vi "initial.vi"(8 "error in (no error)":errorcluster, 11 "ZanCard in":refnum<class "ZanCard.lvclass">) -> (0 "error out":errorcluster, 3 "ZanCard out":refnum<class "ZanCard.lvclass">)   [LabVIEW 2019, in "ZanCard.lvclass"]
uses:
  ZanCard.lvclass
  IOCard.lvclass/IOCard.ctl
  ZanCard.lvclass/ZanCard.ctl
  LLB/zmotion/zaux/zauxdll.lvlib
  IOCard.lvclass
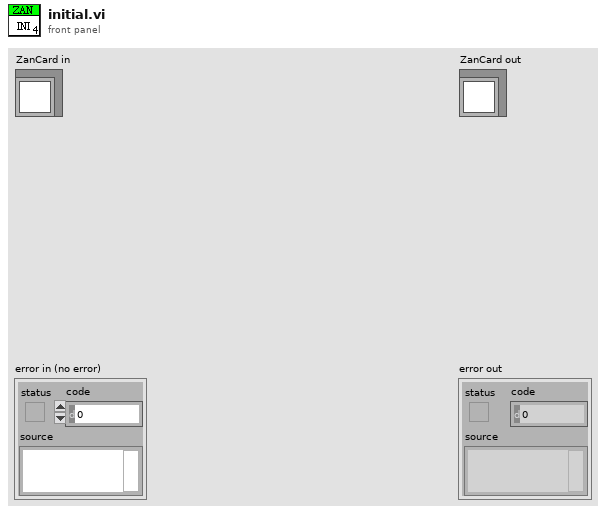
[diagram p1: front panel]
types:
  T1 = typedef "IO Card_Type.ctl" = enum16{"None", "Unidaq32", "6480", "2410C-64", "Zan", "DMC1000B", "16InOut", "Robot", "DMC3600"}
  T2 = cluster{"IO Card Type":T1, "IOType":enum16{"Input", "Output"}, "CardNumber":i32, "ConnectAct":bool, "IP":string}
  T3 = cluster{"CardNumber":i32, "Connect":bool, "Handler":i32}
  T4 = cluster{"Card":i32, "Connect":bool, "Handler":i32}[]
  T5 = cluster{"Card":i32, "Connect":bool, "Handler":i32}
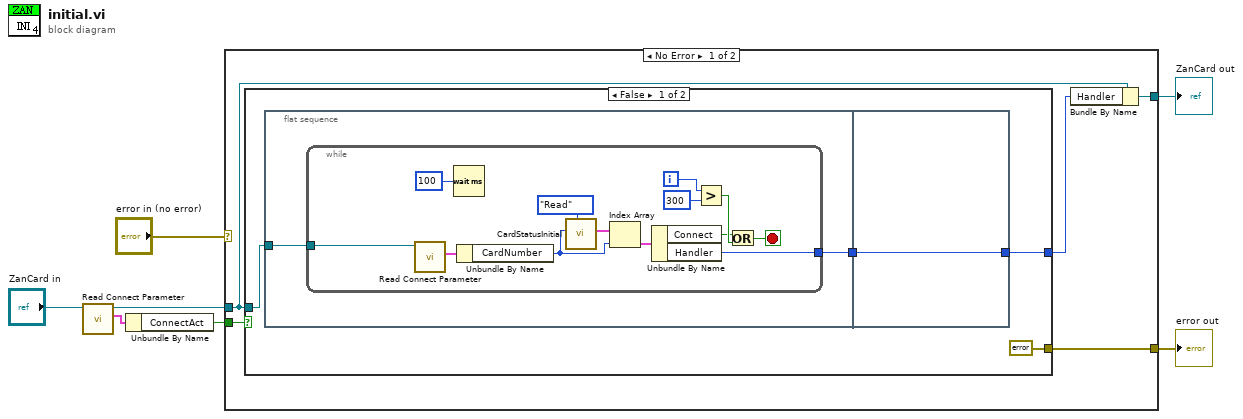
[diagram p0: block diagram]
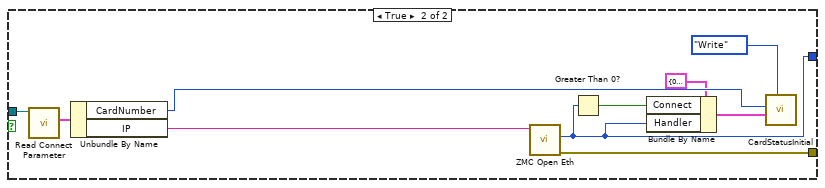
[diagram p2: hidden frame]
diagram:
  n1 = call "Read Connect Parameter.vi"("IOCard in"="ZanCard in") -> ("Connect Parameter"=w2:T2, "IOCard out"=w3:refnum<class "ZanCard.lvclass">)  [unwired: 8 in, 1 out]
  n2 = Unbundle By Name(w2) -> ("ConnectAct"=w1:bool)
  n3 = case shown="No Error" "error in (no error)" {
    selector: "error in (no error)" -> [_ w44]
    tunnel: [w12 w44] -> w6
    tunnel: w3 -> [w9 w43]
    tunnel: [w11 w43] -> w5
    tunnel: w1 -> [w8 _]
    frame No Error {
      n4 = case shown="False" w8 {
        tunnel: [errorcluster {"status"=FALSE, "code"=0, "source"=""} ("error out") w42] -> w12
        tunnel: w9 -> [w14 w41]
        tunnel: [w15 w33] -> w10
        frame False {
          n5 = flat-sequence {
            tunnel: w14 -> [w18]
            tunnel: [w17] -> w13
            tunnel: [w32] -> w15
            tunnel: w13 -> [w32]
            frame #0 {
              n6 = while {
                tunnel: w18 -> [w25]
                tunnel: [w19] -> w17
                i -> [w29]
                stop <- w30 stop-if-true
                n7 = call "Read Connect Parameter.vi"("IOCard in"=w25) -> ("Connect Parameter"=w24:T2)  [unwired: 8 in, 2 out]
                n8 = Wait (ms)(milliseconds to wait=u32 100) -> ()  [unwired: 1 out]
                n9 = Unbundle By Name(w24) -> ("CardNumber"=w22:i32)
                n10 = call "CardStatusInitial.vi"("Action"=enum16{"Initial", "Write", "Read", "Release"}."Read", "CardNumber"=w22) -> ("CardStatus"=w23:T4)  [unwired: 9 in]
                n11 = Index Array(array=w23, index=w22) -> (element=w21:T5)
                n12 = Unbundle By Name(w21) -> ("Connect"=w20:bool, "Handler"=w19:i32)
                n13 = Greater?(x=w29, y=300) -> (0:w27:bool)
                n14 = Or(x=w20, y=w27) -> (x .or. y?=w30:bool)
              }
            }
            frame #1 {
            }
          }
        }
        frame True {
          n15 = call "Read Connect Parameter.vi"("IOCard in"=w41) -> ("Connect Parameter"=w40:T2)  [unwired: 8 in, 2 out]
          n16 = Unbundle By Name(w40) -> ("CardNumber"=w37:i32, "IP"=w39:string)
          n17 = call "ZMC Open Eth.vi"("ipaddr"=w39) -> ("error out"=w42:errorcluster, "phandle out"=w33:u32)  [unwired: 7 in, 2 out]
          n18 = Greater Than 0?(x=w33) -> (x > 0?=w35:bool)
          n19 = Bundle By Name(cluster=T3 {"CardNumber"=0, "Connect"=FALSE, "Handler"=0} ("DataIn"), "Connect"=w35, "Handler"=w33) -> (w34:T3)
          n20 = call "CardStatusInitial.vi"("Action"=enum16{"Initial", "Write", "Read", "Release"}."Write", "DataIn"=w34, "CardNumber"=w37) -> ()  [unwired: 8 in, 1 out]
        }
      }
      n21 = Bundle By Name(cluster=w9, "Handler"=w10) -> (w11:refnum<class "ZanCard.lvclass">)
    }
    frame Error {
    }
  }
  "error out" <- w6
  "ZanCard out" <- w5
